vi "GenerateName.vi"(11 "Configuration":T1) -> (3 "Name":string)   [LabVIEW 2020, in "DependencyViewer.lvlib"]
uses:
  DependencyViewer.lvlib
  DependencyConfiguration.ctl
  FilterOptions.ctl
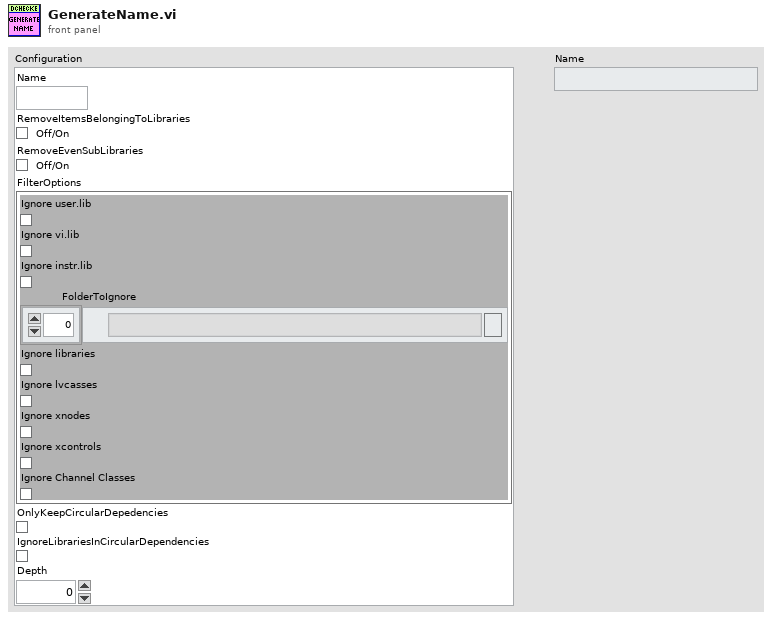
[diagram p1: front panel]
types:
  T1 = typedef "DependencyViewer.lvlib/DependencyConfiguration.ctl" = cluster{"Name":string, "RemoveItemsBelongingToLibraries":bool, "RemoveEvenSubLibraries":bool, "FilterOptions":T2, "OnlyKeepCircularDepedencies":bool, "IgnoreLibrariesInCircularDependencies":bool, "Depth":i32}
  T2 = typedef "DependencyViewer.lvlib/FilterOptions.ctl" = cluster{"Ignore user.lib":bool, "Ignore vi.lib":bool, "Ignore instr.lib":bool, "FolderToIgnore":path[], "Ignore libraries":bool, "Ignore lvcasses":bool, "Ignore xnodes":bool, "Ignore xcontrols":bool, "Ignore Channel Classes":bool}
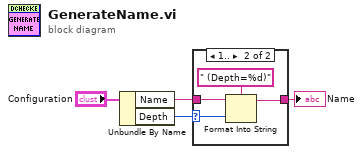
[diagram p0: block diagram]
diagram:
  n1 = Unbundle By Name("Configuration") -> ("Name"=w3:string, "Depth"=w2:i32)
  n2 = case shown="1.." w2 {
    selector: w2 -> [_ w7]
    tunnel: w3 -> [w5 w9]
    tunnel: [w5 w6] -> w4
    frame 0, Default {
    }
    frame 1.. {
      n3 = Format Into String(format string=" (Depth=%d)", initial string=w9, w7) -> (resulting string=w6:string)  [unwired: 1 in, 1 out]
    }
  }
  "Name" <- w4
